vi "getWFMQueue.Initial.vi"(8 "error in (no error)":errorcluster, 11 "DAQmx in":refnum<class "DAQmx.lvclass">) -> (0 "error out":errorcluster, 1 "AO 2":waveform(dbl)[](array[waveform]), 2 "AO 1":waveform(dbl)[](array[waveform]), 3 "DAQmx out":refnum<class "DAQmx.lvclass">)   [LabVIEW 2019, in "DAQmx.lvclass"]
uses:
  DAQmx.lvclass
  DAQmx.lvclass/DAQmx.ctl
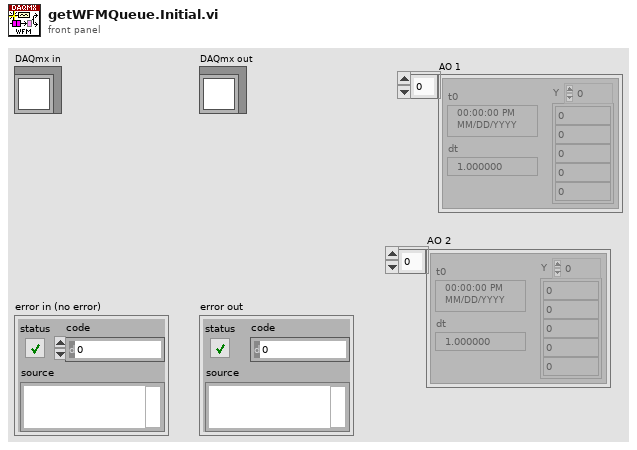
[diagram p1: front panel]
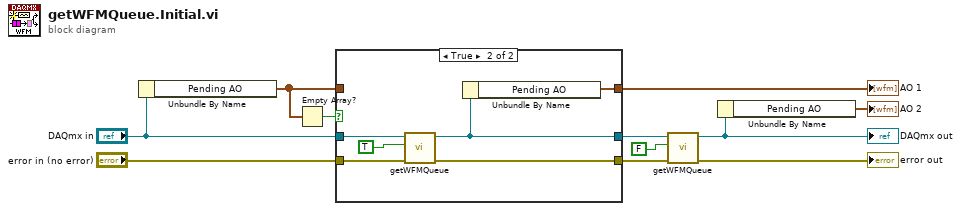
[diagram p0: block diagram]
diagram:
  n1 = Unbundle By Name("DAQmx in") -> ("Pending AO"=w1:waveform(dbl)[])
  n2 = Empty Array?(array=w1) -> (empty?=w2:bool)
  n3 = case shown="True" w2 {
    tunnel: [w13 w16] -> w11
    tunnel: "DAQmx in" -> [w13 w20]
    tunnel: "error in (no error)" -> [w14 w19]
    tunnel: [w12 w15] -> w8
    tunnel: [w14 w18] -> w7
    tunnel: w1 -> [w12 _]
    frame False {
    }
    frame True {
      n4 = call "getWFMQueue.vi"("error in (no error)"=w19, "wait for min buffer?"=TRUE, "DAQmx in"=w20) -> ("error out"=w18:errorcluster, "DAQmx out"=w16:refnum<class "DAQmx.lvclass">)  [unwired: 6 in, 1 out]
      n5 = Unbundle By Name(w16) -> ("Pending AO"=w15:waveform(dbl)[])
    }
  }
  "AO 1" <- w8
  n6 = call "getWFMQueue.vi"("error in (no error)"=w7, "wait for min buffer?"=FALSE, "DAQmx in"=w11) -> ("error out"=→"error out":errorcluster, "DAQmx out"=w4:refnum<class "DAQmx.lvclass">)  [unwired: 6 in, 1 out]
  "DAQmx out" <- w4
  n7 = Unbundle By Name(w4) -> ("Pending AO"=→"AO 2":waveform(dbl)[])
